vi "氨氮插入数据.vi"(0 "table":string, 5 "data":T2={"时间标识"=timestamp(0 s since 1904-01-01), "测量模式"=enum."水样测试", "数据标记表"="N", "监测值"=0.0, "单位"=0, "数据标识"="", "因子编码"=0, "标样参考值"=0.0, "F0"=0.0, "F1"=0.0, "F2"=0.0, "F3"=0.0, "F4"=0.0, "F5"=0.0, "F6"=0.0, "F7"=0.0, "X"=0.0, "温度"=0.0, "湿度"=0.0, "量程标识"="", "SN"=""} {"单位" items=["μg/L", "mg/L", "ppm", "mg/m3", "cm", "ppb", "μg/m3", "%", "nmol/mol", "μmol/mol", "MPN/L", "MPN/100ml", "ng/m3", "NTU", "无量纲", "ms/cm", "μs/cm"]}, 11 "error in (no error)":errorcluster) -> (15 "error out":errorcluster)   [LabVIEW 2016, in "斯坦道氨氮.lvlib"]
uses:
  <vilib>/Utility/sysdir.llb/System Directory Type.ctl
  <vilib>/Utility/error.llb/DialogType.ctl
  <vilib>/addons/database/Auxilliary.llb/DB Tools Column Info.ctl
  <vilib>/addons/database/Auxilliary.llb/DB Tools DataTypes.ctl
  <vilib>/addons/database/Connection.llb/DB Tools Open Connec (String).vi
  <vilib>/addons/database/Connection.llb/Conn Execute.vi
  <vilib>/addons/database/Recordset.llb/Rec Fetch Recordset Data (R).vi
  <vilib>/addons/database/Recordset.llb/Rec Destroy - Connection.vi
  <vilib>/addons/database/NI_Database_API.lvlib
panel:
  out "data输出":T1
  out "为空？":bool
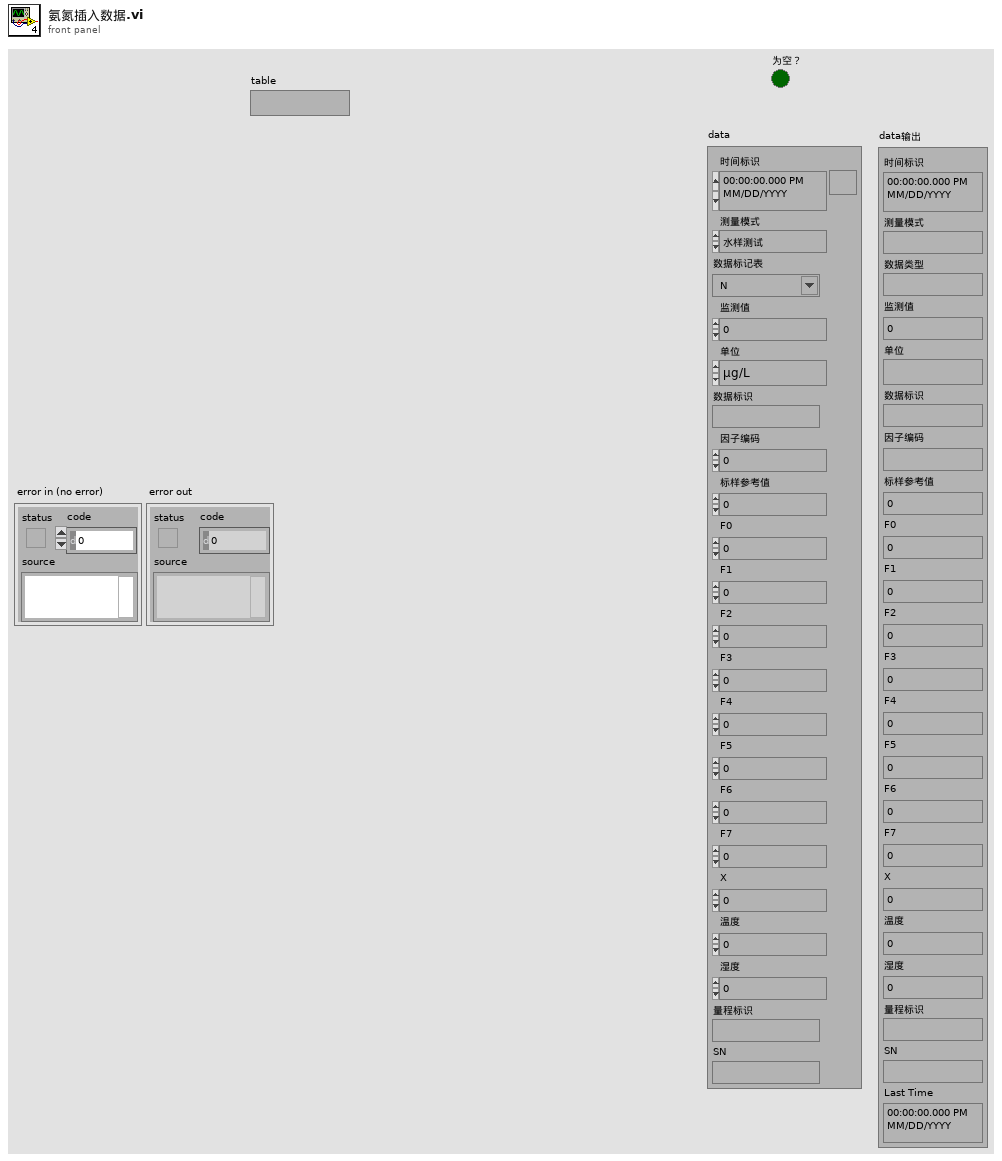
[diagram p1: front panel]
types:
  T1 = cluster{"时间标识":timestamp, "测量模式":string, "数据类型":string, "监测值":sgl, "单位":string, "数据标识":string, "因子编码":string, "标样参考值":sgl, "F0":sgl, "F1":sgl, "F2":sgl, "F3":sgl, "F4":sgl, "F5":sgl, "F6":sgl, "F7":sgl, "X":sgl, "温度":sgl, "湿度":sgl, "量程标识":string, "SN":string, "Last Time":timestamp}
  T2 = cluster{"时间标识":timestamp, "测量模式":enum16{"维护数据", "水样测试", "标样核查", "零点核查", "跨度核查", "空白测试", "平行样测试", "加标回收", "空白校准", "标样校准", "初始化（清洗）"}, "数据标记表":string, "监测值":sgl, "单位":u16, "数据标识":string, "因子编码":u32, "标样参考值":sgl, "F0":sgl, "F1":sgl, "F2":sgl, "F3":sgl, "F4":sgl, "F5":sgl, "F6":sgl, "F7":sgl, "X":sgl, "温度":sgl, "湿度":sgl, "量程标识":string, "SN":string}
  T3 = typedef "DialogType.ctl" = u16
  T4 = typedef "System Directory Type.ctl" = i32
  T5 = typedef "NI_Database_API.lvlib/Conn ObjectReference.ctl" = refnum<k1>
  T6 = typedef "NI_Database_API.lvlib/Rec ObjectReference.ctl" = refnum<k1>
  T7 = typedef "NI_Database_API.lvlib/DB Tools Column Info.ctl" = cluster{"column name":string, "data type":T8, "size":i32, "allow null?":bool}
  T8 = typedef "NI_Database_API.lvlib/DB Tools DataTypes.ctl" = enum16{"String", "Long (I32)", "Single (SGL)", "Double (DBL)", "Date/Time", "Binary"}
  T9 = enum16{"维护数据", "水样测试", "标样核查", "零点核查", "跨度核查", "空白测试", "平行样测试", "加标回收", "空白校准", "标样校准", "初始化（清洗）"}
  T10 = cluster{"测量量程":dbl, "测量精度":dbl, "测量间隔":dbl, "消解温度":dbl, "消解时长":dbl, "空白校准时间":timestamp, "曲线截距":dbl, "曲线斜率":dbl, "测量检出限":dbl, "测量信号值":dbl, "线性相关系数":dbl, "二次多项式系数":dbl, "标样校准时间":timestamp, "稀释倍数":dbl, "三项式系数":dbl, "空白标定系数":dbl, "量程系数":dbl, "F0/ORPA":dbl, "F1/ORPB":dbl, "F2/ORPK":dbl, "F3":dbl, "F4":dbl, "F5":dbl, "F6":dbl, "F7":dbl, "X0/滴定数":dbl, "量程":dbl}
  T11 = cluster{"时间标识":timestamp, "设备":string, "日志信息":string}
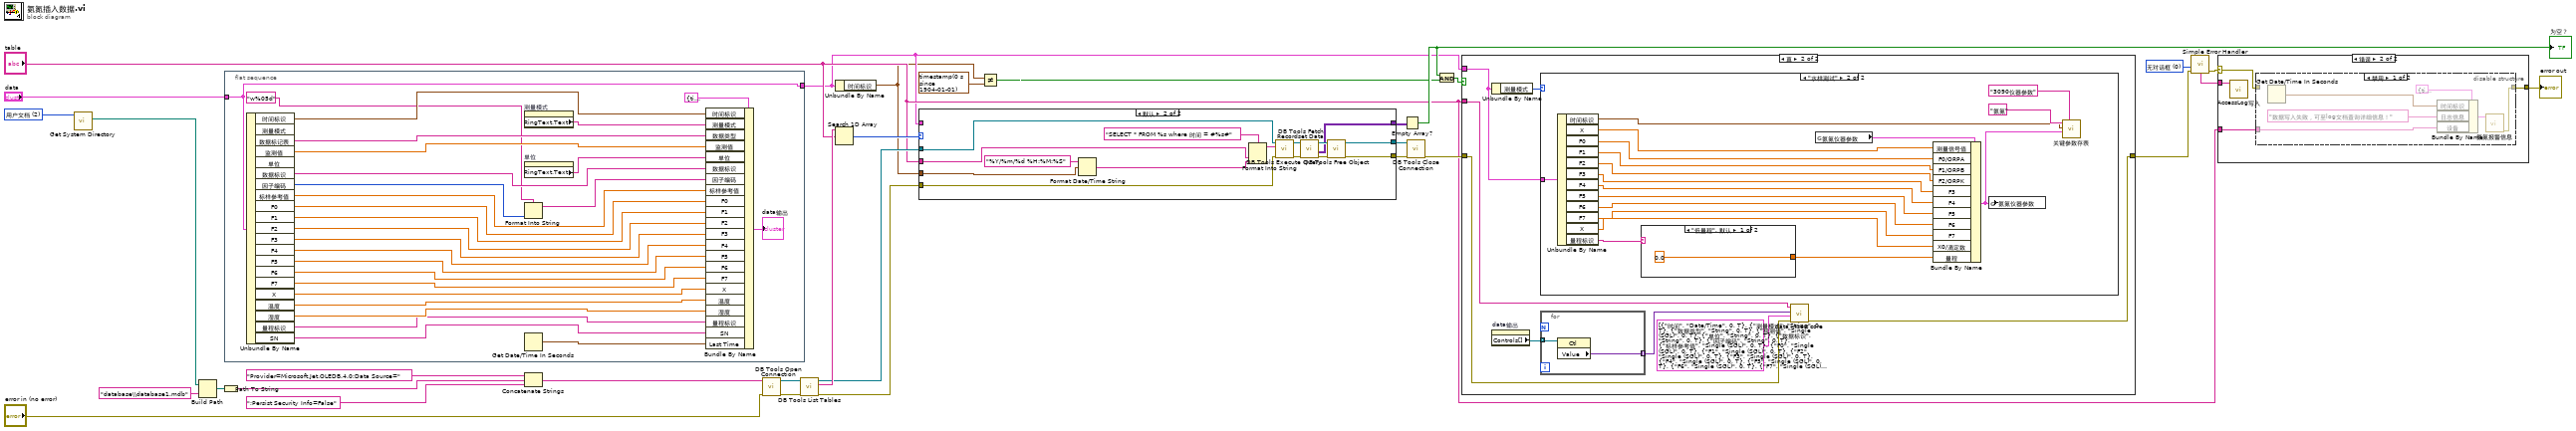
[diagram p0: block diagram]
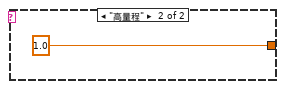
[diagram p6: hidden frame]
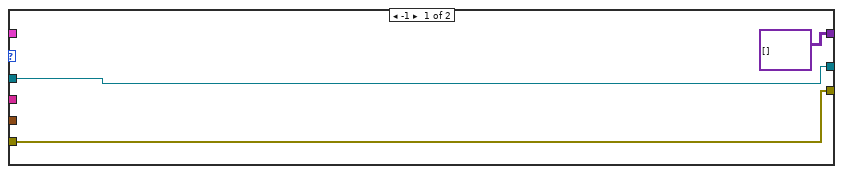
[diagram p7: hidden frame]
diagram:
  w17 = T3 0 items=["无对话框", "确定信息", "继续或停止信息", "确定信息＋警告", "继续/停止+警告"] ("type of dialog (OK msg:1)")
  w32 = T4 2 items=["用户目录"=0, "用户桌面"=1, "用户文档"=2, "用户应用程序数据"=3, "用户设置"=4, "用户临时目录"=5, "公共文档"=6, "公共应用程序数据"=7, "公共设置"=8, "公共缓存"=13, "系统核心库"=9, "系统安装库"=10, "应用程序文件"=11, "启动盘根目录"=12] ("system directory type")
  n1 = call <vilib>:"Get System Directory.vi"("system directory type"=w32) -> ("system directory"=w30:path)  [unwired: 10 in]
  n2 = Build Path(base path=w30, name or relative path="database\\database1.mdb" ("condition")) -> (appended path=w29:path)
  n3 = Path To String(path=w29) -> (string=w28:string)
  n4 = flat-sequence {
    tunnel: "data" -> [w36]
    tunnel: [w36] -> w5
    frame #0 {
      n5 = Unbundle By Name(w36) -> ("时间标识"=w57:timestamp, "数据标记表"=w55:string, "监测值"=w54:sgl, "数据标识"=w52:string, "因子编码"=w35:u32, "标样参考值"=w51:sgl, "F0"=w50:sgl, "F1"=w49:sgl, "F2"=w48:sgl, "F3"=w47:sgl, "F4"=w46:sgl, "F5"=w45:sgl, "F6"=w44:sgl, "F7"=w43:sgl, "X"=w42:sgl, "温度"=w41:sgl, "湿度"=w40:sgl, "量程标识"=w39:string, "SN"=w38:string)  [unwired: 2 out]
      n6 = property on="测量模式" class="Enum (严格)"() -> ("RingText.Text"=w56:string)  [unwired: 2 in, 2 out]
      n7 = property on="单位" class="Ring (严格)"() -> ("RingText.Text"=w53:string)  [unwired: 2 in, 2 out]
      n8 = Format Into String(format string="w%05d" ("格式字符串"), w35) -> (resulting string=w33:string)  [unwired: 2 in, 1 out]
      n9 = Get Date/Time In Seconds() -> (seconds since 1Jan1904=w37:timestamp)
      n10 = Bundle By Name(cluster=T1 {"时间标识"=timestamp(0 s since 1904-01-01), "测量模式"="", "数据类型"="", "监测值"=0.0, "单位"="", "数据标识"="", "因子编码"="", "标样参考值"=0.0, "F0"=0.0, "F1"=0.0, "F2"=0.0, "F3"=0.0, "F4"=0.0, "F5"=0.0, "F6"=0.0, "F7"=0.0, "X"=0.0, "温度"=0.0, "湿度"=0.0, "量程标识"="", "SN"="", "Last Time"=timestamp(0 s since 1904-01-01)} ("data输出"), "时间标识"=w57, "测量模式"=w56, "数据类型"=w55, "监测值"=w54, "单位"=w53, "数据标识"=w52, "因子编码"=w33, "标样参考值"=w51, "F0"=w50, "F1"=w49, "F2"=w48, "F3"=w47, "F4"=w46, "F5"=w45, "F6"=w44, "F7"=w43, "X"=w42, "温度"=w41, "湿度"=w40, "量程标识"=w39, "SN"=w38, "Last Time"=w37) -> (→"data输出":T1)
    }
  }
  n11 = Concatenate Strings("Provider=Microsoft.Jet.OLEDB.4.0;Data Source=" ("condition"), w28, ";Persist Security Info=False" ("condition")) -> (w26:string)
  n12 = call-poly <vilib>:"DB Tools Open Connection.vi"("error in (no error)"="error in (no error)", "connection information"=w26) -> ("error out"=w23:errorcluster, "connection reference"=w24:T5)  [unwired: 6 in]
  n13 = call <vilib>:"DB Tools List Tables.vi"("error in (no error)"=w23, "connection reference"=w24) -> ("error out"=w18:errorcluster, "tables"=w22:string[], "connection reference out"=w19:T5)  [unwired: 3 in]
  n14 = Unbundle By Name(w5) -> ("时间标识"=w3:timestamp)
  n15 = Search 1D Array(1D array=w22, element="table") -> (index of element=w21:i32)  [unwired: 1 in]
  n16 = case shown="默认" w21 {
    tunnel: [variant[][] [] ("recordset data") w73] -> w25
    tunnel: [w62 w72] -> w13
    tunnel: [w61 w71] -> w12
    tunnel: w19 -> [w62 w67]
    tunnel: w18 -> [w61 w66]
    tunnel: "table" -> [_ w64]
    tunnel: w5 -> [_ _]
    tunnel: w3 -> [_ w63]
    frame -1 {
    }
    frame Default {
      n17 = Format Date/Time String(time format string (%c)="%Y/%m/%d %H:%M:%S" ("时间格式字符串(%c)"), seconds (now)=w63) -> (date/time string=w68:string)  [unwired: 1 in]
      n18 = Format Into String(format string="SELECT * FROM %s where 时间 = #%s#" ("格式字符串"), w64, w68) -> (resulting string=w70:string)  [unwired: 2 in, 1 out]
      n19 = call-poly <vilib>:"DB Tools Execute Query.vi"("error in (no error)"=w66, "SQL query"=w70, "connection reference"=w67) -> ("error out"=w74:errorcluster, "recordset reference"=w77:T6)  [unwired: 5 in]
      n20 = call-poly <vilib>:"DB Tools Fetch Recordset Data.vi"("error in (no error)"=w74, "recordset reference"=w77) -> ("error out"=w75:errorcluster, "recordset data"=w73:variant[][], "recordset reference out"=w76:T6)  [unwired: 3 in]
      n21 = call-poly <vilib>:"DB Tools Free Object.vi"("error in (no error)"=w75, "recordset reference"=w76) -> ("error out"=w71:errorcluster, "connection reference"=w72:T5)  [unwired: 8 in]
    }
  }
  n22 = Not Equal?(x=w3, y=timestamp(0 s since 1904-01-01)) -> (x != y?=w1:bool)
  n23 = Empty Array?(array=w25) -> (empty?=w20:bool)
  "为空？" <- w20
  n24 = call <vilib>:"DB Tools Close Connection.vi"("error in (no error)"=w12, "connection reference"=w13) -> ("error out"=w9:errorcluster)  [unwired: 5 in]
  n25 = And(x=w20, y=w1) -> (x .and. y?=w2:bool)
  n26 = case shown="真" w2 {
    tunnel: "table" -> [_ w79]
    tunnel: w5 -> [_ w81]
    tunnel: w9 -> [w78 w82]
    tunnel: [w78 w83] -> w8
    frame False {
    }
    frame True {
      n27 = Unbundle By Name(w81) -> ("测量模式"=w80:T9)
      n28 = property on="data输出" class="Clust (严格)"() -> ("Controls[]"=w84:refnum<vi>[])  [unwired: 2 in, 2 out]
      n29 = case shown="\"水样测试\"" w80 {
        tunnel: w81 -> [_ w103]
        frame "维护数据", Default {
        }
        frame "水样测试" {
          n30 = Unbundle By Name(w103) -> ("时间标识"=w102:timestamp, "X"=w101:sgl, "F0"=w89:sgl, "F1"=w90:sgl, "F2"=w91:sgl, "F3"=w92:sgl, "F4"=w93:sgl, "F5"=w94:sgl, "F6"=w95:sgl, "F7"=w96:sgl, "X"=w97:sgl, "量程标识"=w99:string)
          n31 = case shown="\"低量程\", 默认" w99 {
            tunnel: [0.0 ("量程") 1.0 ("量程")] -> w98
            frame "低量程", Default {
            }
            frame "高量程" {
            }
          }
          n32 = global read "氨氮断电保存全局变量.vi" "氨氮仪器参数"() -> (w106:T10)
          n33 = Bundle By Name(cluster=w106, "测量信号值"=w101, "F0/ORPA"=w89, "F1/ORPB"=w90, "F2/ORPK"=w91, "F3"=w92, "F4"=w93, "F5"=w94, "F6"=w95, "F7"=w96, "X0/滴定数"=w97, "量程"=w98) -> (w104:T10)
          n34 = global write "氨氮断电保存全局变量.vi" "氨氮仪器参数"(w104) -> ()
          n35 = call "关键参数存表.vi"("table"="3090仪器参数", "仪器参数"=w104, "datatime"=w102, "仪器名称"="氨氮") -> ()  [unwired: 7 in, 1 out]
        }
      }
      n36 = for {
        tunnel: w84 -> [w88] mode=indexing
        tunnel: [w87] -> w85 mode=indexing
        n37 = property class="Ctl"(reference=w88) -> ("Value"=w87:variant)  [unwired: 1 in, 2 out]
      }
      n38 = call "data insert core.vi"("error in (no error)"=w82, "column information"=T7[] [{"column name"="时间", "data type"=enum."Date/Time", "size"=0, "allow null?"=TRUE}, {"column name"="测量模式", "data type"=enum."String", "size"=0, "allow null?"=TRUE}, {"column name"="数据类型", "data type"=enum."String", "size"=0, "allow null?"=TRUE}, {"column name"="检测值", "data type"=enum."Single (SGL)", "size"=0, "allow null?"=TRUE}, {"column name"="单位", "data type"=enum."String", "size"=0, "allow null?"=TRUE}, {"column name"="数据标识", "data type"=enum."String", "size"=0, "allow null?"=TRUE}, {"column name"="因子编码", "data type"=enum."String", "size"=0, "allow null?"=TRUE}, {"column name"="标样参考值", "data type"=enum."Single (SGL)", "size"=0, "allow null?"=TRUE}, {"column name"="F0", "data type"=enum."Single (SGL)", "size"=0, "allow null?"=TRUE}, {"column name"="F1", "data type"=enum."Single (SGL)", "size"=0, "allow null?"=TRUE}, {"column name"="F2", "data type"=enum."Single (SGL)", "size"=0, "allow null?"=TRUE}, {"column name"="F3", "data type"=enum."Single (SGL)", "size"=0, "allow null?"=TRUE}, {"column name"="F4", "data type"=enum."Single (SGL)", "size"=0, "allow null?"=TRUE}, {"column name"="F5", "data type"=enum."Single (SGL)", "size"=0, "allow null?"=TRUE}, {"column name"="F6", "data type"=enum."Single (SGL)", "size"=0, "allow null?"=TRUE}, {"column name"="F7", "data type"=enum."Single (SGL)", "size"=0, "allow null?"=TRUE}, {"column name"="X", "data type"=enum."Single (SGL)", "size"=0, "allow null?"=TRUE}, {"column name"="温度", "data type"=enum."Single (SGL)", "size"=0, "allow null?"=TRUE}, {"column name"="湿度", "data type"=enum."Single (SGL)", "size"=0, "allow null?"=TRUE}, {"column name"="量程标识", "data type"=enum."String", "size"=0, "allow null?"=TRUE}, {"column name"="SN", "data type"=enum."String", "size"=0, "allow null?"=TRUE}, {"column name"="LastTime", "data type"=enum."Date/Time", "size"=0, "allow null?"=TRUE}], "data"=w85, "table"=w79) -> ("error out"=w83:errorcluster)  [unwired: 7 in]
    }
  }
  n39 = call <vilib>:"Simple Error Handler.vi"("type of dialog (OK msg:1)"=w17, "error in (no error)"=w8) -> ("error out"=w16:errorcluster, "message"=w15:string)  [unwired: 3 in, 3 out]
  n40 = case shown="错误" w16 {
    selector: w16 -> [_ w109]
    tunnel: w15 -> [_ w110]
    tunnel: [_ w112] -> w14
    tunnel: "table" -> [_ w111]
    frame No Error {
    }
    frame Error {
      n41 = call "AccessLog写入.vi"("Log"=w110) -> ()  [unwired: 11 in]
      n42 = disable-structure shown="禁用" {
        disable-tunnel: [w116 w119] -> w112
        disable-tunnel: w111 -> [w114 _]
        disable-tunnel: w109 -> [_ w119]
        frame Disabled {
          n43 = Get Date/Time In Seconds() -> (seconds since 1Jan1904=w115:timestamp)
          n44 = Bundle By Name(cluster=T11 {"时间标识"=timestamp(0 s since 1904-01-01), "设备"="", "日志信息"=""} ("data in"), "时间标识"=w115, "日志信息"="数据写入失败，可至log文档查询详细信息！", "设备"=w114) -> (w117:T11)
          n45 = call "氨氮报警信息.vi"("data in"=w117) -> ("error out"=w116:errorcluster)  [unwired: 10 in]
        }
        frame Enabled {
        }
      }
    }
  }
  "error out" <- w14
